vi "GloToBDD.vi"() -> ()   [LabVIEW 2020]
uses:
  <vilib>/Utility/error.llb/whitespace.ctl
panel:
  out "error out":errorcluster
  out "requette":string
  out "Array 2":string[](array[string])
  out "Array":string[](array[string])
  in  "errin":errorcluster
  # "2023-01-09 16:50:38"
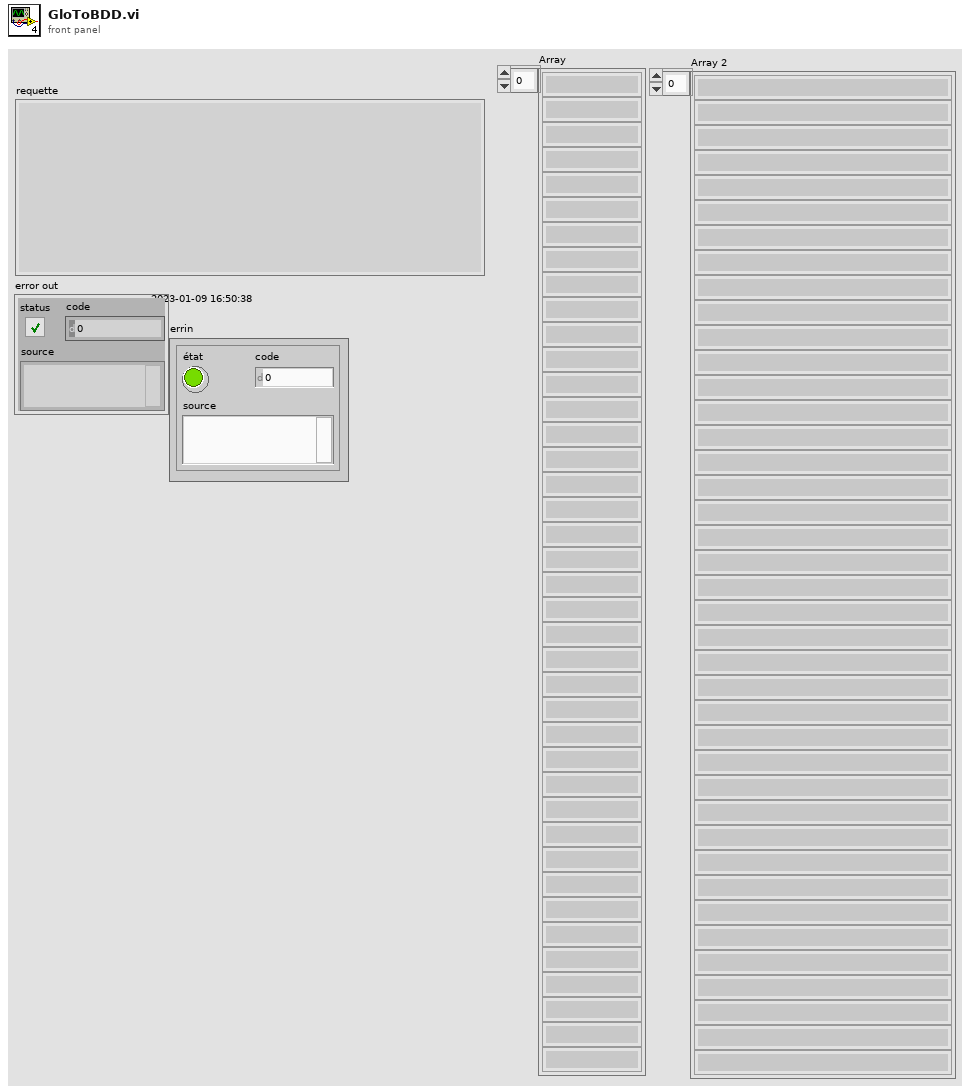
[diagram p1: front panel]
types:
  T1 = typedef "whitespace.ctl" = u16
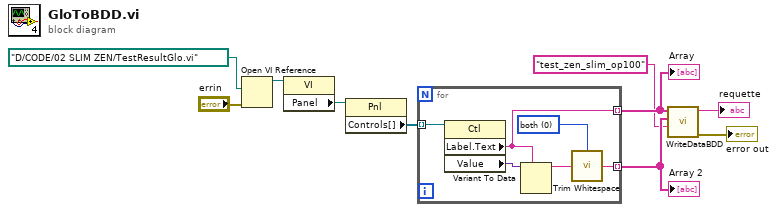
[diagram p0: block diagram]
diagram:
  n1 = Open VI Reference(vi path=path "D:/CODE/02 SLIM ZEN/TestResultGlo.vi", error in (no error)="errin") -> (vi reference=w8:refnum<vi>)  [unwired: 4 in, 1 out]
  n2 = property class="VI"(reference=w8) -> ("Panel"=w7:refnum<vi>)  [unwired: 1 in, 2 out]
  n3 = property class="Pnl"(reference=w7) -> ("Controls[]"=w6:refnum<vi>[])  [unwired: 1 in, 2 out]
  n4 = for {
    tunnel: w6 -> [w16] mode=indexing
    tunnel: [w14] -> w5 mode=indexing
    tunnel: [w12] -> w4 mode=indexing
    w11 = T1 0 items=["both", "start of string", "end of string"] ("location (both)")
    n5 = property class="Ctl"(reference=w16) -> ("Label.Text"=w14:string, "Value"=w15:variant)  [unwired: 1 in, 2 out]
    n6 = Variant To Data(type=w14, Variant=w15) -> (data=w13:string)  [unwired: 1 in, 1 out]
    n7 = call <vilib>:"Trim Whitespace.vi"("string"=w13, "location (both)"=w11) -> ("trimmed string"=w12:string)
  }
  "Array" <- w5
  "Array 2" <- w4
  n8 = call "WriteDataBDD.vi"("table"="test_zen_slim_op100", "data"=w4, "id"=w5) -> ("error out"=→"error out":errorcluster, "requette"=→"requette":string)  [unwired: 7 in]
